vi "Garage Door.vi"() -> ()   [LabVIEW 2012]
panel:
  in  "?":bool
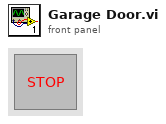
[diagram p1: front panel]
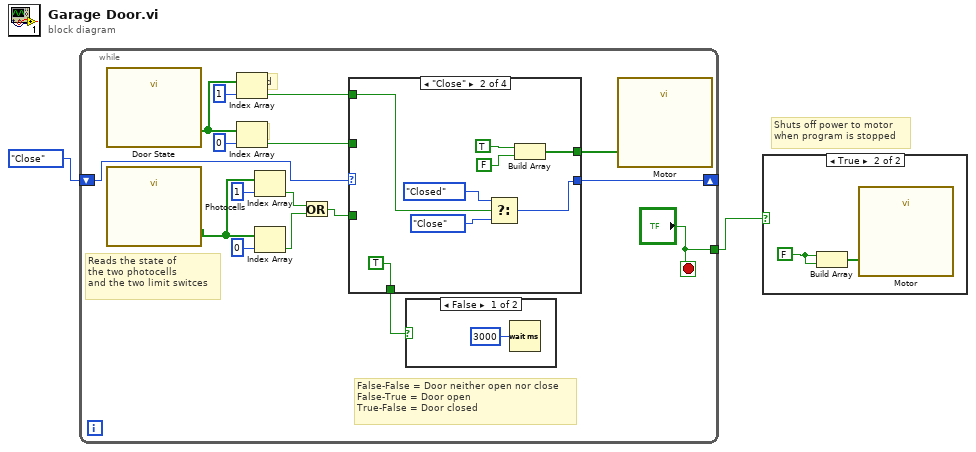
[diagram p0: block diagram]
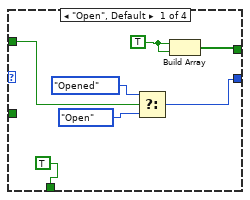
[diagram p4: hidden frame]
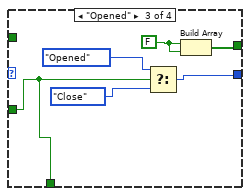
[diagram p5: hidden frame]
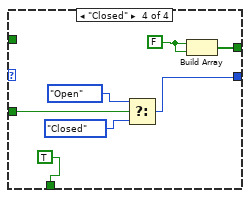
[diagram p6: hidden frame]
diagram:
  # "Shuts off power to motor\nwhen program is stopped"
  n1 = while {
    tunnel: ["?"] -> w1
    shift-right: [w6] -> _
    shift-left: enum16{"Open", "Close", "Opened", "Closed"}."Close" -> [w8]
    stop <- "?" stop-if-true
    # "False-False = Door neither open nor close\nFalse-True = Door open\nTrue-False = Door closed"
    # "Reads the state of \nthe two photocells\nand the two limit switces"
    # "Open"
    # "Closed"
    n2 = call "Door State"() -> ("data"=w16:bool[])  [unwired: 17 in, 2 out]
    n3 = call "Photocells"() -> ("data"=w13:bool[])  [unwired: 17 in, 2 out]
    n4 = Index Array(array=w16, index=1) -> (element=w4:bool)
    n5 = Index Array(array=w16, index=0) -> (element=w5:bool)
    n6 = Index Array(array=w13, index=1) -> (element=w12:bool)
    n7 = Index Array(array=w13, index=0) -> (element=w11:bool)
    n8 = Or(x=w12, y=w11) -> (x .or. y?=w7:bool)
    n9 = case shown="\"Close\"" w8 {
      tunnel: [w25 w32 w39 w46] -> w9
      tunnel: w7 -> [_ _ w36 w45]
      tunnel: [w21 w28 w37 w42] -> w6
      tunnel: w5 -> [w24 _ _ _]
      tunnel: w4 -> [_ w29 _ _]
      tunnel: [TRUE TRUE w36 TRUE] -> w3
      frame "Open", Default {
        w26 = TRUE
        n10 = Select(t=enum16{"Open", "Close", "Opened", "Closed"}."Opened", s=w24, f=enum16{"Open", "Close", "Opened", "Closed"}."Open") -> (s? t:f=w21:enum16{"Open", "Close", "Opened", "Closed"})
        n11 = Build Array(w26, w26) -> (w25:bool[])
      }
      frame "Close" {
        n12 = Select(t=enum16{"Open", "Close", "Opened", "Closed"}."Closed", s=w29, f=enum16{"Open", "Close", "Opened", "Closed"}."Close") -> (s? t:f=w28:enum16{"Open", "Close", "Opened", "Closed"})
        n13 = Build Array(TRUE, FALSE) -> (w32:bool[])
      }
      frame "Opened" {
        w40 = FALSE
        n14 = Select(t=enum16{"Open", "Close", "Opened", "Closed"}."Opened", s=w36, f=enum16{"Open", "Close", "Opened", "Closed"}."Close") -> (s? t:f=w37:enum16{"Open", "Close", "Opened", "Closed"})
        n15 = Build Array(w40, w40) -> (w39:bool[])
      }
      frame "Closed" {
        w47 = FALSE
        n16 = Select(t=enum16{"Open", "Close", "Opened", "Closed"}."Open", s=w45, f=enum16{"Open", "Close", "Opened", "Closed"}."Closed") -> (s? t:f=w42:enum16{"Open", "Close", "Opened", "Closed"})
        n17 = Build Array(w47, w47) -> (w46:bool[])
      }
    }
    n18 = case shown="False" w3 {
      frame False {
        n19 = Wait (ms)(milliseconds to wait=u32 3000) -> ()  [unwired: 1 out]
      }
      frame True {
      }
    }
    n20 = call "Motor"("data"=w9) -> ()  [unwired: 17 in, 2 out]
  }
  n21 = case shown="True" w1 {
    frame False {
    }
    frame True {
      w49 = FALSE
      n22 = Build Array(w49, w49) -> (w48:bool[])
      n23 = call "Motor"("data"=w48) -> ()  [unwired: 17 in, 2 out]
    }
  }
